vi "Call Function with I32 Python Objects.vi"(8 "error in (no error)":errorcluster) -> (0 "error out":errorcluster)   [LabVIEW 2020]
uses:
  G-Embedded-Python-Interpreter-Toolkit/Call.vi
  G-Embedded-Python-Interpreter-Toolkit/Null Py Object Refnum.vi
  G-Embedded-Python-Interpreter-Toolkit/Merge Call Library Errors.vi
  <vilib>/addons/_JKI Toolkits/Caraya/classes/Assert/Assert Not Error.vi
  <vilib>/addons/_JKI Toolkits/Caraya/classes/Assert/Assert Equal Value and Type_Variant.vi
  G-Embedded-Python-Interpreter-Toolkit/G-Embedded-Python-Interpreter-Toolkit.lvlib
  <vilib>/addons/_JKI Toolkits/Caraya/classes/Test/Test.lvclass
  <vilib>/addons/_JKI Toolkits/Caraya/classes/Assert/Assert.lvclass
panel:
  out "Value":i32
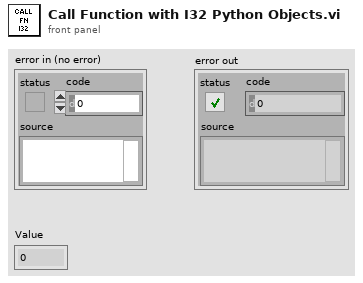
[diagram p1: front panel]
types:
  T1 = typedef "G-Embedded-Python-Interpreter-Toolkit.lvlib/Python Object Reference.ctl" = refnum<k1>
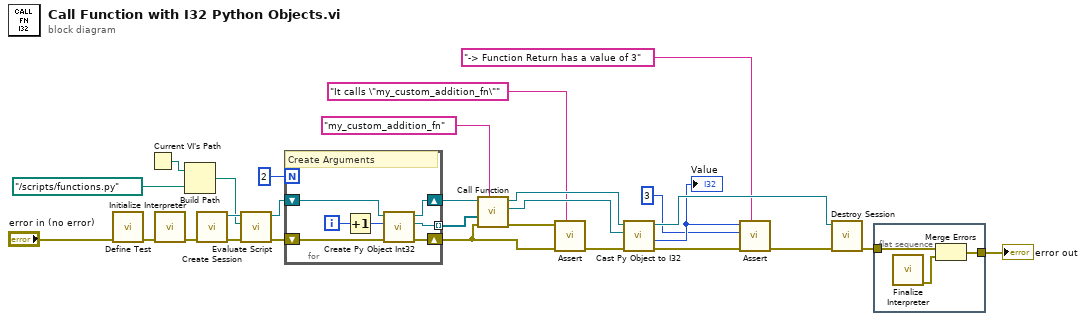
[diagram p0: block diagram]
diagram:
  n1 = call <vilib>:"Define Test.vi"("error in (no error)"="error in (no error)") -> ("error out"=w28:errorcluster)  [unwired: 10 in]
  n2 = Current VI's Path() -> (path=w23:path)
  n3 = call "Initialize Interpreter.vi"("error in (no error)"=w28) -> ("error out"=w25:errorcluster)  [unwired: 9 in, 1 out]
  n4 = Build Path(base path=w23, name or relative path=path "../scripts/functions.py" ("Path")) -> (appended path=w21:path)
  n5 = call "Create Session.vi"("error in (no error)"=w25) -> ("error out"=w20:errorcluster, "Session Handle"=w24:refnum<data-value>)  [unwired: 9 in]
  n6 = call "Evaluate Script.vi"("error in (no error)"=w20, "Script File Path"=w21, "Session Handle in"=w24) -> ("error out"=w17:errorcluster, "Session Handle out"=w18:refnum<data-value>)  [unwired: 7 in]
  n7 = for {
    N: 2 -> [_]
    shift-right: [w31] -> w16
    shift-left: w18 -> [w35]
    shift-right: [w32] -> w5
    shift-left: w17 -> [w34]
    tunnel: [w30] -> w15 mode=indexing
    i -> [w33]
    # "Create Arguments"
    n8 = Increment(x=w33) -> (x+1=w29:i32)
    n9 = call "Create Py Object Int32.vi"("error in (no error)"=w34, "Value"=w29, "Session Handle in"=w35) -> ("error out"=w32:errorcluster, "Python Object Refnum"=w30:T1, "Session Handle out"=w31:refnum<data-value>)  [unwired: 6 in]
  }
  n10 = call "Call Function.vi"("Function Name"="my_custom_addition_fn", "error in (no error)"=w5, "Arguments (Default -Empty)"=w15, "Data Value Reference in"=w16) -> ("error out"=w4:errorcluster, "Returned Python Object Refnum"=w13:T1, "Data Value Reference out"=w14:refnum<data-value>)  [unwired: 5 in]
  n11 = call-poly <vilib>:"Assert.vi"("Label"="It calls \"my_custom_addition_fn\"", "error in (no error)"=w5, "Not Error?"=w4) -> ("error out"=w3:errorcluster)  [unwired: 8 in]
  n12 = call "Cast Py Object to I32.vi"("error in (no error)"=w3, "Python Object Refnum in"=w13, "Session Handle in"=w14) -> ("error out"=w2:errorcluster, "Value"=w10:i32, "Session Handle out"=w12:refnum<data-value>)  [unwired: 5 in, 1 out]
  "Value" <- w10
  n13 = call-poly <vilib>:"Assert.vi"("Label"="-> Function Return has a value of 3", "error in (no error)"=w2, "Y"=3 ("Value"), "X"=w10) -> ("error out"=w9:errorcluster)  [unwired: 7 in]
  n14 = call "Destroy Session.vi"("error in (no error)"=w9, "Session Handle"=w12) -> ("error out"=w19:errorcluster)  [unwired: 9 in]
  n15 = flat-sequence {
    tunnel: w19 -> [w38]
    tunnel: [w36] -> w26
    frame #0 {
      n16 = call "Finalize Interpreter.vi"() -> ("error out"=w37:errorcluster)  [unwired: 11 in]
      n17 = Merge Errors(w38, w37) -> (w36:errorcluster)
    }
  }
  "error out" <- w26
